vi "Cursor Move.vi"(0 "3D Plot.lvclass in":refnum<class "3D Plot.lvclass">, 1 "Coords":cluster{"Horizontal":i32, "Vertical":i32}, 2 "Control Ref Queue":T16, 3 "Actual Transform In":T1, 5 "Object Cluster In":T15, 7 "Cursor ID In":i32, 9 "Tracking Cursor?":bool, 11 "error in (no error)":errorcluster, 12 "Multiplot Represention":T3) -> (4 "3D Plot.lvclass out":refnum<class "3D Plot.lvclass">, 6 "Object Cluster Out":T15, 8 "Cursor ID":i32, 10 "Drag Cursor?":bool, 13 "Update Plot?":bool, 14 "Cursor Property Array":T6, 15 "error out":errorcluster)   [LabVIEW 2020, in "3D Plot.lvclass"]
uses:
  3D Plot.lvclass
  3DMathPlot Ctrl Act Queue.ctl
  3DMathPlot Ctrl Act Cluster.ctl
  3DMathPlot State Class.ctl
  Object Cluster.ctl
  Cursor Property Array.ctl
  Cursor Property.ctl
  Cursor Position.ctl
  Cursor Point.ctl
  Sprite Type.ctl
  Cursor Line.ctl
  Line Type.ctl
  Cursor Plane.ctl
  Cursor Text.ctl
  Multiplot Representation.ctl
  Plot Representation.ctl
  Range Clusters.ctl
  Mesh Data.ctl
  Actual Transform.ctl
  3D Plot.lvclass/3D Plot.ctl
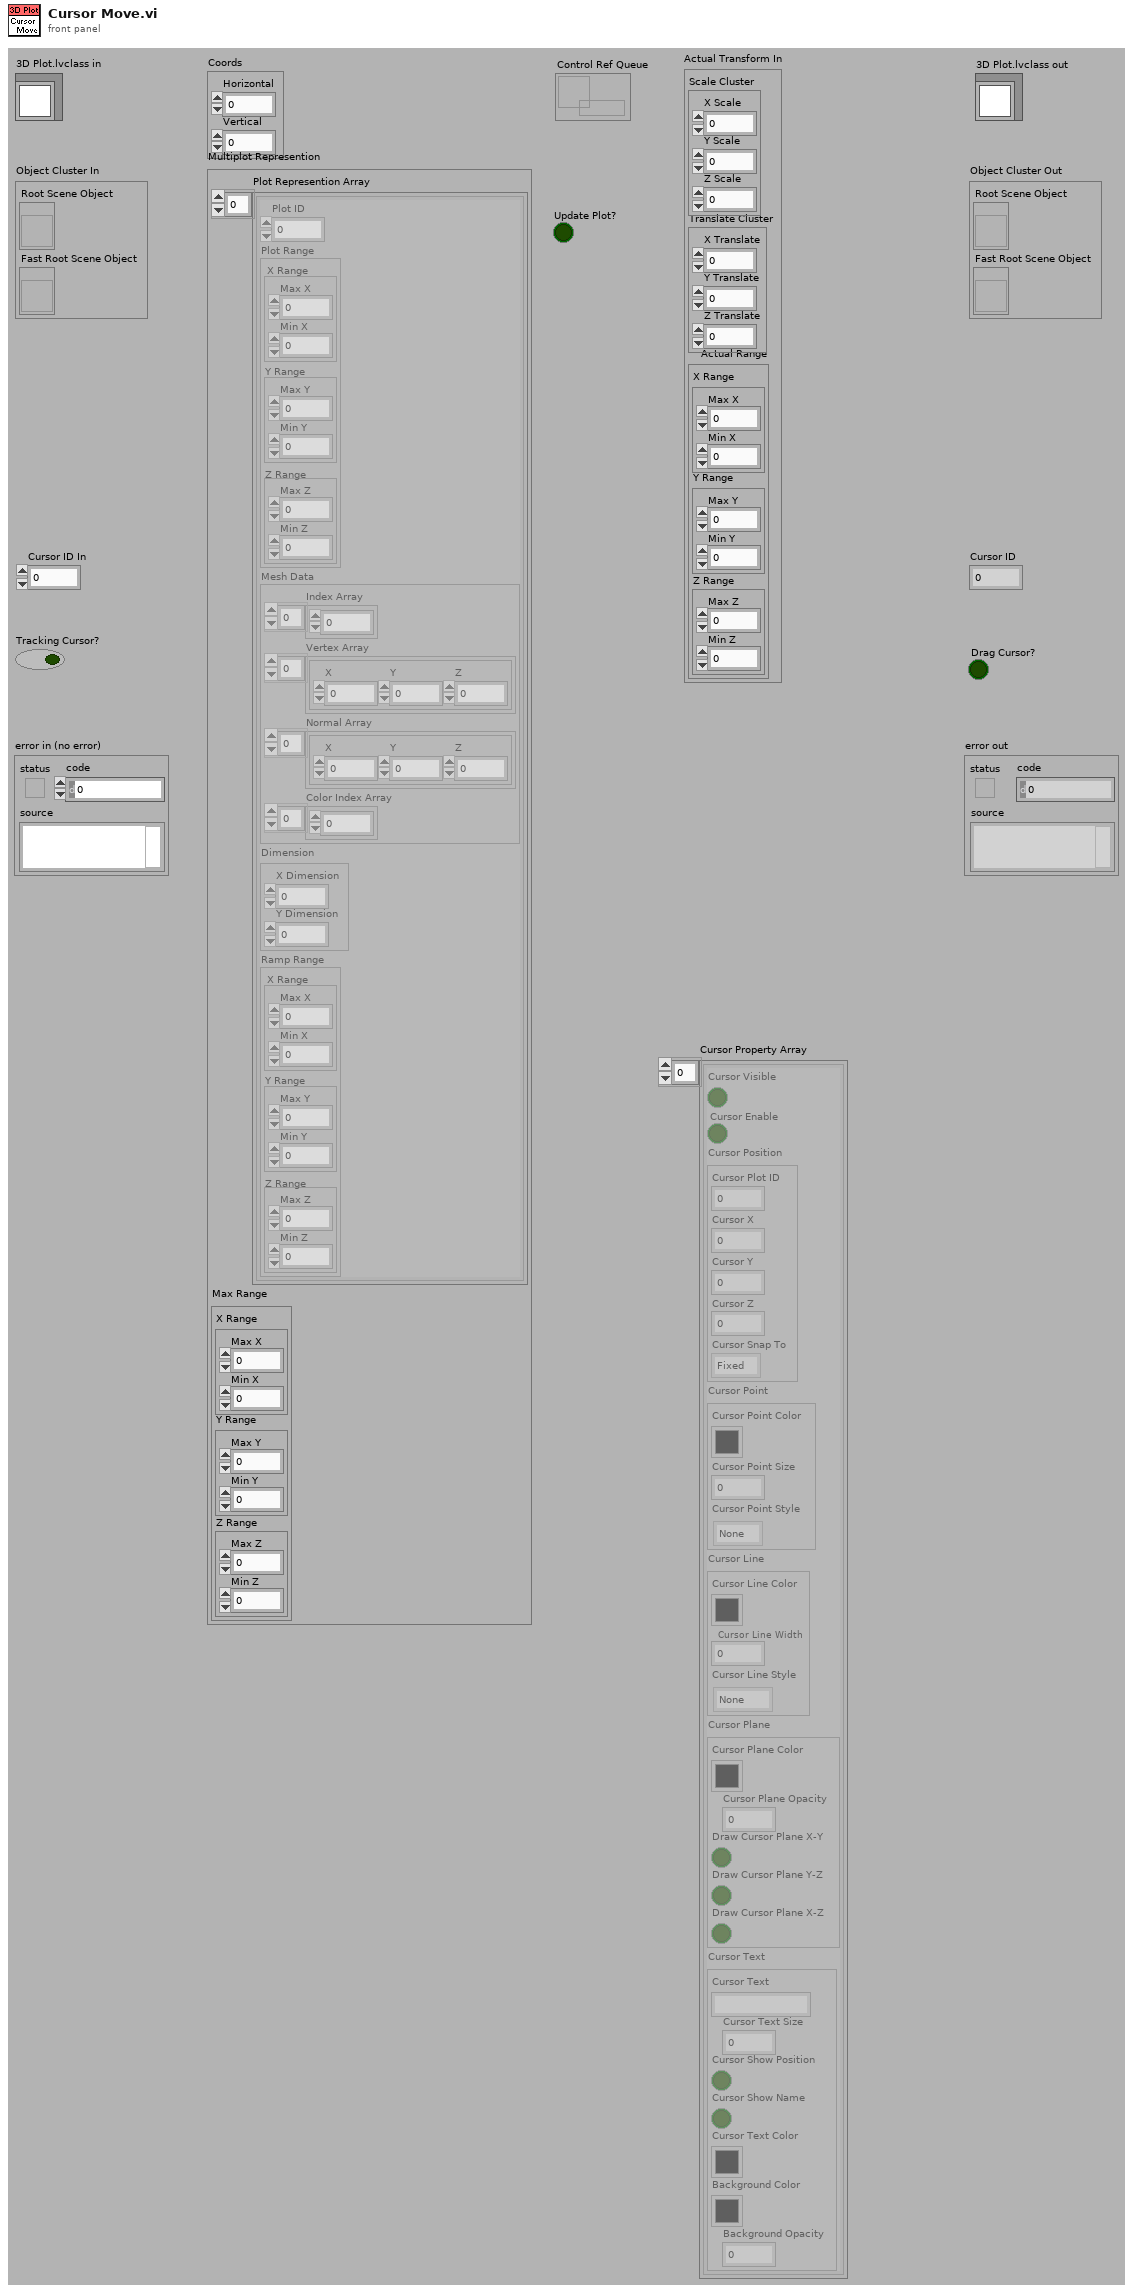
[diagram p1: front panel]
types:
  T1 = typedef "3D Plot.lvclass/Actual Transform.ctl" = cluster{"Scale Cluster":cluster{"X Scale":sgl, "Y Scale":sgl, "Z Scale":sgl}, "Translate Cluster":cluster{"X Translate":sgl, "Y Translate":sgl, "Z Translate":sgl}, "Actual Range":T2}
  T2 = typedef "3D Plot.lvclass/Range Clusters.ctl" = cluster{"X Range":cluster{"Max X":sgl, "Min X":sgl}, "Y Range":cluster{"Max Y":sgl, "Min Y":sgl}, "Z Range":cluster{"Max Z":sgl, "Min Z":sgl}}
  T3 = typedef "3D Plot.lvclass/Multiplot Representation.ctl" = cluster{"Plot Represention Array":T4[], "Max Range":T2}
  T4 = typedef "3D Plot.lvclass/Plot Representation.ctl" = cluster{"Plot ID":i32, "Plot Range":T2, "Mesh Data":T5, "Dimension":cluster{"X Dimension":i32, "Y Dimension":i32}, "Ramp Range":T2}
  T5 = typedef "3D Plot.lvclass/Mesh Data.ctl" = cluster{"Index Array":u32[], "Vertex Array":cluster{"X":sgl, "Y":sgl, "Z":sgl}[], "Normal Array":cluster{"X":sgl, "Y":sgl, "Z":sgl}[], "Color Index Array":i32[]}
  T6 = typedef "3D Plot.lvclass/Cursor Property Array.ctl" = T7[]
  T7 = typedef "3D Plot.lvclass/Cursor Property.ctl" = cluster{"Cursor Visible":bool, "Cursor Enable":bool, "Cursor Position":T8, "Cursor Point":T9, "Cursor Line":T11, "Cursor Plane":T13, "Cursor Text":T14}
  T8 = typedef "3D Plot.lvclass/Cursor Position.ctl" = cluster{"Cursor Plot ID":i32, "Cursor X":sgl, "Cursor Y":sgl, "Cursor Z":sgl, "Cursor Snap To":enum16{"Fixed", "Nearest Plot", "Snap to Plot"}}
  T9 = typedef "3D Plot.lvclass/Cursor Point.ctl" = cluster{"Cursor Point Color":u32, "Cursor Point Size":sgl, "Cursor Point Style":T10}
  T10 = typedef "3D Plot.lvclass/Sprite Type.ctl" = enum16{"None", "Empty Square", "Solid Square", "Empty Diamond", "Solid Diamond", "Empty Circle", "Solid Circle", "Asterisk", "Bold X", "Wireframe Sphere", "Solid Sphere", "Wireframe Cube", "Solid Cube"}
  T11 = typedef "3D Plot.lvclass/Cursor Line.ctl" = cluster{"Cursor Line Color":u32, "Cursor Line Width":sgl, "Cursor Line Style":T12}
  T12 = typedef "3D Plot.lvclass/Line Type.ctl" = enum16{"None", "Solid", "Dash", "Dot", "Dash Dot"}
  T13 = typedef "3D Plot.lvclass/Cursor Plane.ctl" = cluster{"Cursor Plane Color":u32, "Cursor Plane Opacity":sgl, "Draw Cursor Plane X-Z":bool, "Draw Cursor Plane Y-Z":bool, "Draw Cursor Plane X-Y":bool}
  T14 = typedef "3D Plot.lvclass/Cursor Text.ctl" = cluster{"Cursor Text":string, "Cursor Text Size":u16, "Cursor Show Position":bool, "Cursor Show Name":bool, "Cursor Text Color":u32, "Background Color":u32, "Background Opacity":sgl}
  T15 = typedef "3D Plot.lvclass/Object Cluster.ctl" = cluster{"Root Scene Object":refnum<vi>, "Fast Root Scene Object":refnum<vi>}
  T16 = typedef "3DMathPlot Ctrl Act Queue.ctl" = refnum<queue>
  T17 = typedef "3DMathPlot Ctrl Act Cluster.ctl" = cluster{"3D Picture Control":refnum<vi>, "Render Window Refnum":refnum<vi>, "XY Graph":refnum<vi>, "Intensity Graph":refnum<vi>, "Color Legend Palette":refnum<vi>, "Projection Palette":refnum<vi>, "XControl  Ref":refnum<vi>, "Facade Ref":refnum<vi>, "Export Image Ref":refnum<vi>, "Clear Data Flag":bool, "Display State Change Class":T18}
  T18 = typedef "3DMathPlot State Class.ctl" = enum16{"Update All Objects (Undo)", "Update Light Object Only", "Update Axis Object Only", "Update Plot Object Only", "Update Cursor Object Only", "Update Axis Plot Cursor Objects", "No Update"}
  T19 = enum32{"Towards X-Y Plane", "Towards X-Z Plane", "Towards Y-Z Plane", "User Defined"}
  T20 = enum16{"None", "Spherical", "Flying", "Oriented"}
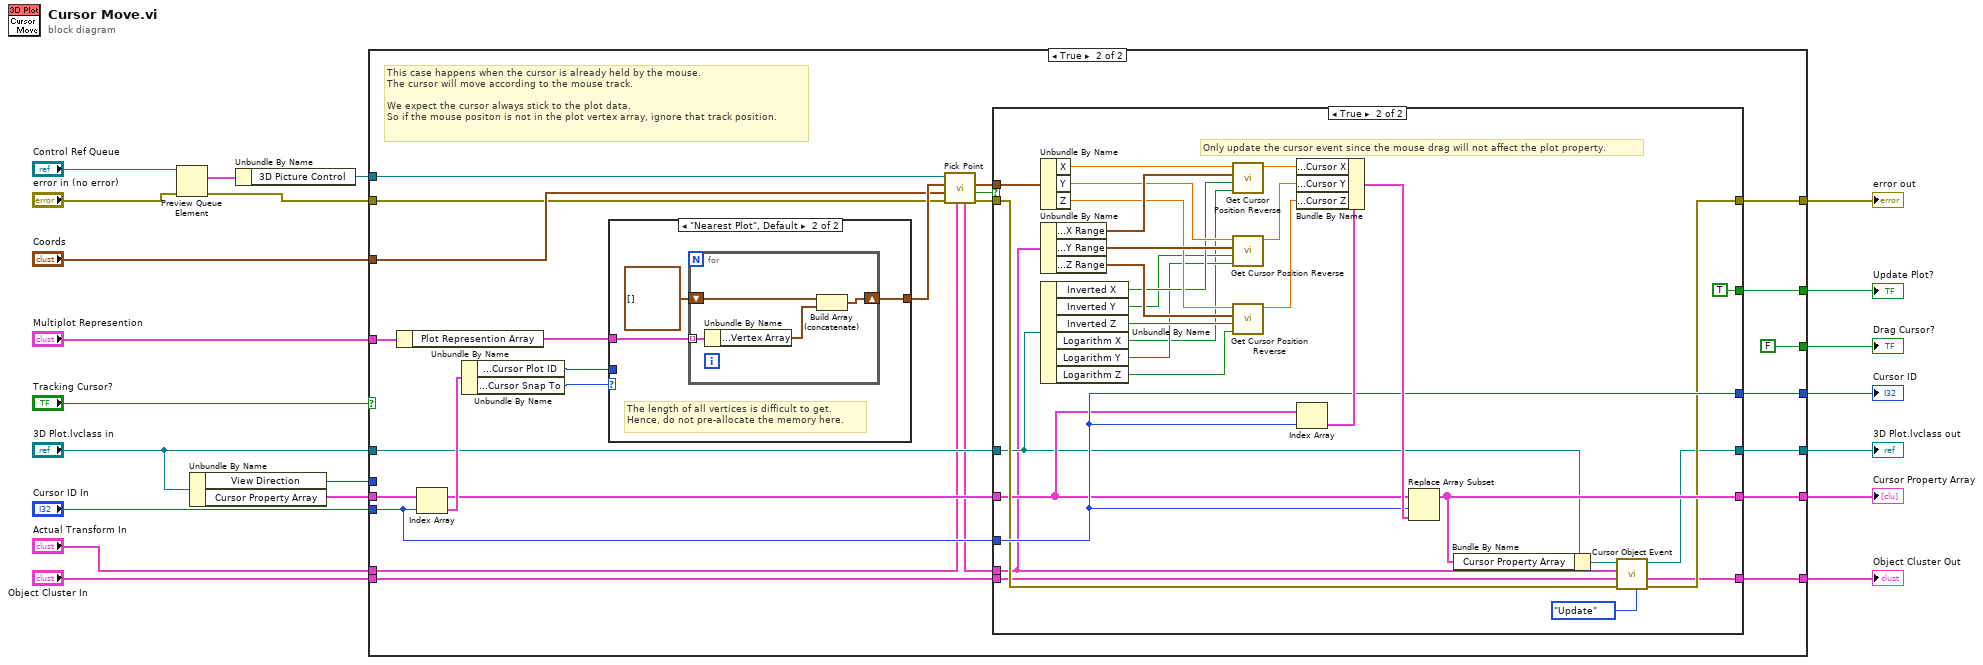
[diagram p0: block diagram]
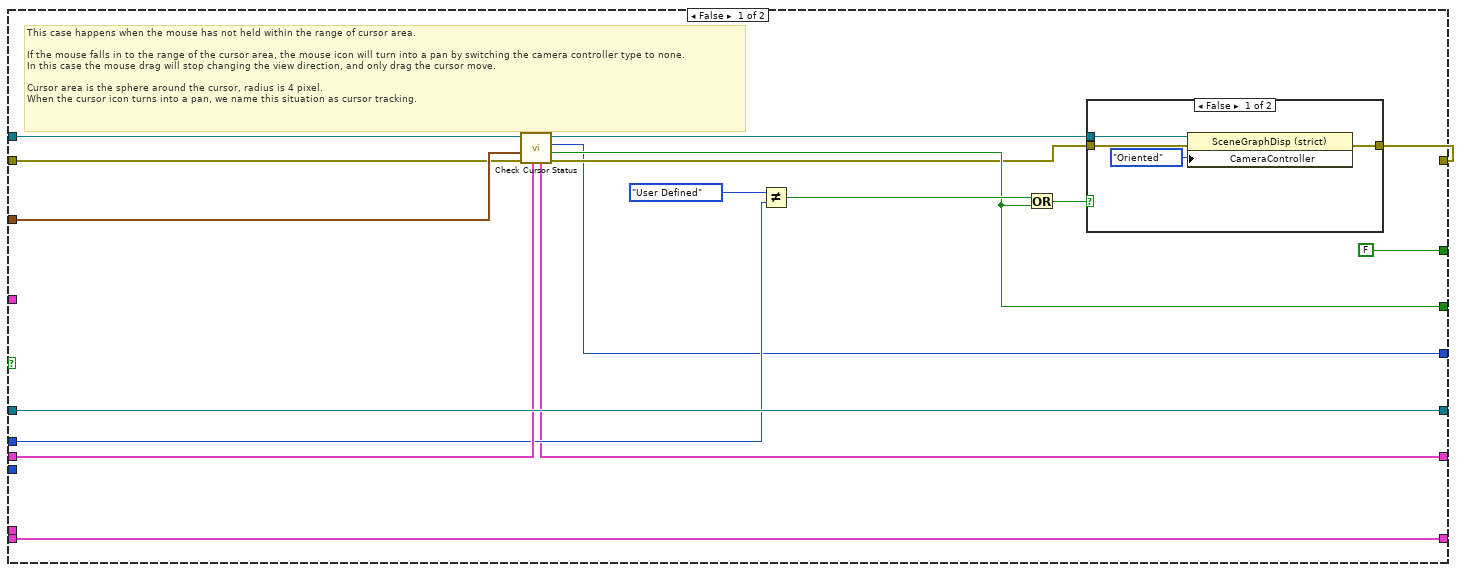
[diagram p2: hidden frame]
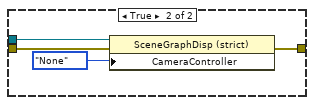
[diagram p3: hidden frame]
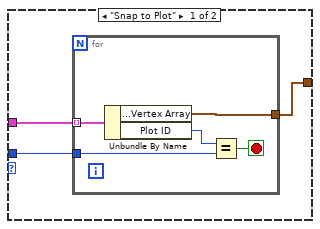
[diagram p4: hidden frame]
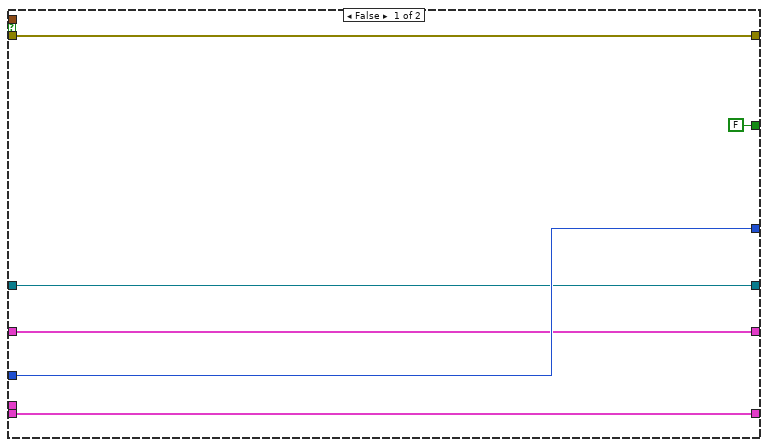
[diagram p5: hidden frame]
diagram:
  n1 = Preview Queue Element(queue="Control Ref Queue", error in (no error)="error in (no error)") -> (element=w5:T17, error out=w1:errorcluster)  [unwired: 3 out]
  n2 = Unbundle By Name("3D Plot.lvclass in") -> ("View Direction"=w3:T19, "Cursor Property Array"=w4:T6)
  n3 = Unbundle By Name(w5) -> ("3D Picture Control"=w2:refnum<vi>)
  n4 = case shown="True" "Tracking Cursor?" {
    tunnel: "Coords" -> [w32 w54]
    tunnel: "3D Plot.lvclass in" -> [w31 w58]
    tunnel: "Cursor ID In" -> [_ w61]
    tunnel: "Object Cluster In" -> [w38 w71]
    tunnel: [w38 w70] -> w18
    tunnel: [w33 FALSE ("Drag Cursor?")] -> w19
    tunnel: [w24 w56] -> w6
    tunnel: "Actual Transform In" -> [_ w49]
    tunnel: w2 -> [w28 w53]
    tunnel: w1 -> [w26 w51]
    tunnel: [w35 w68] -> w16
    tunnel: [FALSE ("Drag Cursor?") w67] -> w15
    tunnel: [w23 w66] -> w14
    tunnel: [w31 w64] -> w12
    tunnel: "Multiplot Represention" -> [_ w63]
    tunnel: w4 -> [w30 w57]
    tunnel: w3 -> [w29 _]
    frame False {
      # "This case happens when the mouse has not held within the range of cursor area.\n\nIf the mouse falls in to the range of the cursor area, the mouse icon will turn into a pan by switching the camera controller type to none. \nIn this case the mouse drag will stop changing the view direction, and only drag the cursor move.\n\nCursor area is the sphere around the cursor, radius is 4 pixel.\nWhen the cursor icon turns into a pan, we name this situation as cursor tracking."
      n5 = call "Check Cursor Status.vi"("Cursor Property Array In"=w30, "error in (no error)"=w26, "Coords"=w32, "3D Picture Control In"=w28) -> ("error out"=w25:errorcluster, "Drag Cursor?"=w33:bool, "Cursor ID"=w24:i32, "3D Picture Control Out"=w27:refnum<vi>, "Cursor Property Array Out"=w23:T6)  [unwired: 3 in]
      n6 = Not Equal?(x=T19."User Defined" ("y"), y=w29) -> (x != y?=w37:bool)
      n7 = Or(x=w37, y=w33) -> (x .or. y?=w36:bool)
      n8 = case shown="False" w36 {
        tunnel: w27 -> [w42 w46]
        tunnel: w25 -> [w41 w45]
        tunnel: [w40 w44] -> w35
        frame False {
          n9 = property on="Property Node" class="SceneGraphDisp (strict)"(reference=w42, error in=w41, "CameraController"=T20."Oriented" ("Camera Controller:Type")) -> (error out=w40:errorcluster)  [unwired: 1 out]
        }
        frame True {
          n10 = property on="Property Node" class="SceneGraphDisp (strict)"(reference=w46, error in=w45, "CameraController"=T20."None" ("Camera Controller:Type")) -> (error out=w44:errorcluster)  [unwired: 1 out]
        }
      }
    }
    frame True {
      # "This case happens when the cursor is already held by the mouse.\nThe cursor will move according to the mouse track.\n\nWe expect the cursor always stick to the plot data.\nSo if the mouse positon is not in the plot vertex array, ignore that track position."
      n11 = Unbundle By Name(w63) -> ("Plot Represention Array"=w62:T4[])
      n12 = Index Array(array=w57, index=w61) -> (element=w60:T7)
      n13 = Unbundle By Name(w60) -> ("Cursor Position.Cursor Plot ID"=w59:i32, "Cursor Position.Cursor Snap To"=w47:enum16{"Fixed", "Nearest Plot", "Snap to Plot"})
      n14 = case shown="\"Nearest Plot\", Default" w47 {
        tunnel: w62 -> [w74 w82]
        tunnel: [w72 w81] -> w55
        tunnel: w59 -> [w73 _]
        frame "Snap to Plot" {
          n15 = for {
            tunnel: w74 -> [w78] mode=indexing
            tunnel: w73 -> [w79]
            tunnel: [w77] -> w72
            stop <- w76 stop-if-true
            n16 = Unbundle By Name(w78) -> ("Mesh Data.Vertex Array"=w77:cluster{"X":sgl, "Y":sgl, "Z":sgl}[], "Plot ID"=w75:i32)
            n17 = Equal?(x=w75, y=w79) -> (x = y?=w76:bool)
          }
        }
        frame "Nearest Plot", Default {
          # "The length of all vertices is difficult to get. \nHence, do not pre-allocate the memory here."
          n18 = for {
            tunnel: w82 -> [w86] mode=indexing
            shift-right: [w84] -> w81
            shift-left: cluster{"X":sgl, "Y":sgl, "Z":sgl}[] [] -> [w83]
            n19 = Unbundle By Name(w86) -> ("Mesh Data.Vertex Array"=w85:cluster{"X":sgl, "Y":sgl, "Z":sgl}[])
            n20 = Build Array (concatenate)(w83, w85) -> (w84:cluster{"X":sgl, "Y":sgl, "Z":sgl}[])
          }
        }
      }
      n21 = call "Pick Point.vi"("Actual Transform In"=w49, "error in (no error)"=w51, "Coords"=w54, "Vertex Array"=w55, "3D Picture Control In"=w53) -> ("error out"=w50:errorcluster, "Hit Any Point?"=w52:bool, "Snap Cursor Position"=w65:cluster{"X":sgl, "Y":sgl, "Z":sgl}, "Actual Transform Out"=w48:T1)  [unwired: 2 in, 1 out]
      n22 = case shown="True" w52 {
        tunnel: w58 -> [w88 w109]
        tunnel: w61 -> [w91 w120]
        tunnel: w65 -> [_ w122]
        tunnel: w71 -> [w92 w114]
        tunnel: [w92 w113] -> w70
        tunnel: [w91 w120] -> w56
        tunnel: [w90 w116] -> w68
        tunnel: w50 -> [w90 w117]
        tunnel: [FALSE ("Drag Cursor?") TRUE ("Drag Cursor?")] -> w67
        tunnel: [w87 w118] -> w66
        tunnel: [w88 w115] -> w64
        tunnel: w48 -> [_ w108]
        tunnel: w57 -> [w87 w110]
        frame False {
        }
        frame True {
          # "Only update the cursor event since the mouse drag will not affect the plot property."
          n23 = Unbundle By Name(w122) -> ("X"=w104:sgl, "Y"=w103:sgl, "Z"=w102:sgl)
          n24 = Unbundle By Name(w108) -> ("Actual Range.X Range"=w107:cluster{"Max X":sgl, "Min X":sgl}, "Actual Range.Y Range"=w106:cluster{"Max Y":sgl, "Min Y":sgl}, "Actual Range.Z Range"=w105:cluster{"Max Z":sgl, "Min Z":sgl})
          n25 = Unbundle By Name(w109) -> ("Inverted X"=w98:bool, "Inverted Y"=w97:bool, "Inverted Z"=w96:bool, "Logarithm X"=w93:bool, "Logarithm Y"=w94:bool, "Logarithm Z"=w95:bool)
          n26 = call "Get Cursor Position Reverse.vi"("Logarithm?"=w93, "Inverted?"=w98, "Range"=w107, "Cursor Value In"=w104) -> ("Cursor Value Out"=w99:sgl)  [unwired: 7 in]
          n27 = call "Get Cursor Position Reverse.vi"("Logarithm?"=w94, "Inverted?"=w97, "Range"=w106, "Cursor Value In"=w103) -> ("Cursor Value Out"=w100:sgl)  [unwired: 7 in]
          n28 = call "Get Cursor Position Reverse.vi"("Logarithm?"=w95, "Inverted?"=w96, "Range"=w105, "Cursor Value In"=w102) -> ("Cursor Value Out"=w101:sgl)  [unwired: 7 in]
          n29 = Index Array(array=w110, index=w120) -> (element=w123:T7)
          n30 = Bundle By Name(cluster=w123, "Cursor Position.Cursor X"=w99, "Cursor Position.Cursor Y"=w100, "Cursor Position.Cursor Z"=w101) -> (w121:T7)
          n31 = Replace Array Subset(array=w110, new element=w121, index=w120) -> (w118:T6)
          n32 = Bundle By Name(cluster=w109, "Cursor Property Array"=w118) -> (w112:refnum<class "3D Plot.lvclass">)
          n33 = call "Cursor Object Event.vi"("Cursor Action"=enum16{"Update", "Remove", "Nothing"}."Update", "error in (no error)"=w117, "Object Cluster In"=w114, "Actual Transform In"=w108, "3D Plot.lvclass in"=w112) -> ("error out"=w116:errorcluster, "Object Cluster Out"=w113:T15, "3D Plot.lvclass out"=w115:refnum<class "3D Plot.lvclass">)  [unwired: 2 in, 2 out]
        }
      }
    }
  }
  "Cursor ID" <- w6
  "Drag Cursor?" <- w19
  "error out" <- w16
  "Update Plot?" <- w15
  "Object Cluster Out" <- w18
  "Cursor Property Array" <- w14
  "3D Plot.lvclass out" <- w12
